vi "Events.vi"(11 "Control Event Registrations in":refnum<class "Control Event Registrations.lvclass">) -> (2 "Events":T1[](array[typedef]))   [LabVIEW 2020, in "VolatusGUI.lvlib" / "Control Event Registrations.lvclass"]
uses:
  Control Event Registrations.lvclass
  Event Registration.ctl
  Control Event.ctl
  Control Event Registrations.lvclass/Control Event Registrations.ctl
  VolatusGUI.lvlib
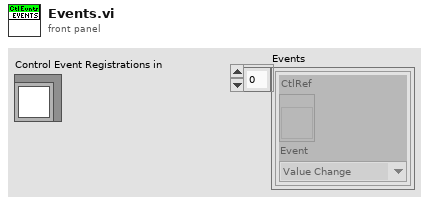
[diagram p1: front panel]
types:
  T1 = typedef "VolatusGUI.lvlib/Event Registration.ctl" = cluster{"CtlRef":refnum<vi>, "Event":T2}
  T2 = typedef "VolatusGUI.lvlib/Control Event.ctl" = enum16{"Value Change", "Shortcut Menu", "Mouse Down"}
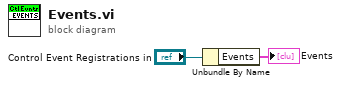
[diagram p0: block diagram]
diagram:
  n1 = Unbundle By Name("Control Event Registrations in") -> ("Events"=→"Events":T1[])
